vi "Get Payload File Path.vi"(8 "error in":errorcluster, 11 "custom device ref in":T1 format="%.0x") -> (0 "error out":errorcluster, 1 "MD5 checksum":string, 2 "frame array file path":path, 3 "custom device ref out":T1 format="%.0x", 4 "found file?":bool, 6 "found Tx Gen?":bool)   [LabVIEW 2020, in "AIM ARINC 664 Scripting.lvlib"]
uses:
  AIM ARINC 664 Scripting.lvlib
  <vilib>/NI VeriStand/Custom Device API/Custom Device Item Ref.ctl
  Constants.vi
  <vilib>/NI VeriStand/Custom Device Tools/Custom Device Utility Library/NI VeriStand - Search for Item by GUID.vi
  <vilib>/NI VeriStand/Custom Device API/Get Item Property (Dependent File).vi
  <vilib>/NI VeriStand/Custom Device API/Custom Device API.lvlib
  <vilib>/NI VeriStand/Custom Device Tools/Custom Device Utility Library/Custom Device Utility Library.lvlib
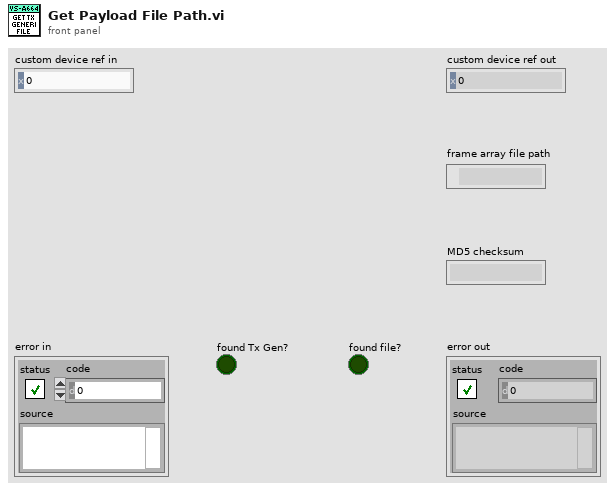
[diagram p1: front panel]
types:
  T1 = typedef "Custom Device API.lvlib/Custom Device Item Ref.ctl" = u64
  T2 = typedef "Custom Device API.lvlib/Dependent File Optional Info.ctl" = cluster{"Version":string, "RTDestination":path, "ForceDownload":bool, "SupportedTarget":string, "MD5":string}
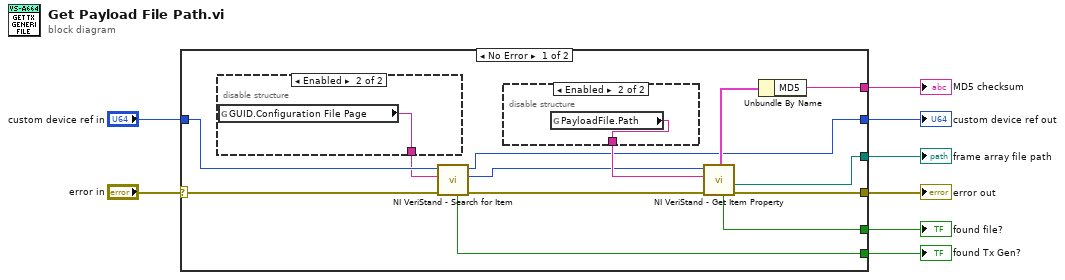
[diagram p0: block diagram]
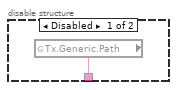
[diagram p2: hidden frame]
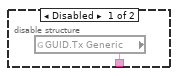
[diagram p3: hidden frame]
diagram:
  n1 = case shown="No Error" "error in" {
    selector: "error in" -> [w14 w27]
    tunnel: "custom device ref in" -> [w19 w26]
    tunnel: [w21 w27] -> w7
    tunnel: [w10 w26] -> w6
    tunnel: [w18 _] -> w4
    tunnel: [w17 _] -> w3
    tunnel: [w15 _] -> w2
    tunnel: [w9 _] -> w1
    frame No Error {
      n2 = disable-structure shown="Enabled" {
        disable-tunnel: [w24 w25] -> w12
        frame Disabled {
          n3 = global read "Constants.vi" "GUID.Tx Generic"() -> (w24:string)
        }
        frame Enabled {
          n4 = global read "Constants.vi" "GUID.Configuration File Page"() -> (w25:string)
        }
      }
      n5 = call-poly <vilib>:"NI VeriStand - Search for Item.vi"("error in"=w14, "Item GUID"=w12, "Section Ref in"=w19) -> ("error out"=w13:errorcluster, "Item Ref"=w11:T1, "Section Ref out"=w10:T1, "Found"=w9:bool)  [unwired: 5 in]
      n6 = disable-structure shown="Enabled" {
        disable-tunnel: [w22 w23] -> w20
        frame Disabled {
          n7 = global read "Constants.vi" "Tx.Generic.Path"() -> (w22:string)
        }
        frame Enabled {
          n8 = global read "Constants.vi" "PayloadFile.Path"() -> (w23:string)
        }
      }
      n9 = call-poly <vilib>:"NI VeriStand - Get Item Property.vi"("error in (no error)"=w13, "Property Name"=w20, "Item Ref in"=w11) -> ("error out"=w21:errorcluster, "Path"=w18:path, "Found"=w17:bool, "OptionalInfo"=w16:T2)  [unwired: 4 in, 1 out]
      n10 = Unbundle By Name(w16) -> ("MD5"=w15:string)
    }
    frame Error {
    }
  }
  "error out" <- w7
  "frame array file path" <- w4
  "custom device ref out" <- w6
  "found file?" <- w3
  "MD5 checksum" <- w2
  "found Tx Gen?" <- w1
